vi "OAT Even Angle Signal Subset (1 Channel).vi"(0 "even-angle signal":cluster{"r0":dbl, "dr":dbl, "Y":dbl[]}={"r0"=0.0, "dr"=1.0, "Y"=[]} {"r0" format="%.2p"; "dr" format="%.2p"; "Y" format="%.2f"}, 5 "even-angle channel info":T1={"channel name"="", "description"="", " channel info"={"sensor sensitivity"=1000.0, "engineering units"=1, "dB reference"=1.0, "custom label"="EU", "weighting filter"=0, "pregain"=0.0}} {"channel info"."pregain" format="%.2f"; "channel info"."weighting filter" items=["Linear", "A-weighting", "B-weighting", "C-weighting", "ITU-R 468-4", "Dolby", "CCITT", "C-message", "Wb", "Wc", "Wd", "We", "Wf", "Wh", "Wj", "Wk", "Wm", "AES17 20 kHz lowpass", "AES17 40 kHz lowpass", "AES17 20 kHz highpass", "AES17 40 kHz highpass"]; "channel info"."dB reference" format="%^.1e"; "channel info"."engineering units" items=["custom..."=0, "V"=1, "A"=21, "C"=30, "pC"=31, "s"=32, "-"=29, "Pa"=2, "N"=20, "g"=3, "m/s^2"=4, "m/s"=5, "m"=6, "mm/s"=12, "mm"=13, "micron/s"=14, "micron"=15, "in/s^2"=7, "in/s"=8, "in"=9, "mil/s"=10, "mil"=11, "rad/s^2"=16, "rad/s"=17, "rad"=18, "deg/s^2"=26, "deg/s"=27, "deg"=28, "RPM"=22, "cycle/s^2"=23, "Hz"=24, "cycle"=25, "strain"=19]; "channel info"."sensor sensitivity" format="%#_5f"}, 7 "start [rev]":dbl format="%0.2f", 9 "duration [rev]":dbl=1.0 format="%0.2f", 11 "error in (no error)":errorcluster) -> (4 "even-angle signal subset":cluster{"r0":dbl, "dr":dbl, "Y":dbl[]}={"r0"=0.0, "dr"=1.0, "Y"=[]} {"r0" format="%.2p"; "dr" format="%.2p"; "Y" format="%.2f"}, 6 "even-angle channel info":T1={"channel name"="", "description"="", " channel info"={"sensor sensitivity"=1000.0, "engineering units"=1, "dB reference"=1.0, "custom label"="EU", "weighting filter"=0, "pregain"=0.0}} {"channel info"."pregain" format="%.2f"; "channel info"."weighting filter" items=["Linear", "A-weighting", "B-weighting", "C-weighting", "ITU-R 468-4", "Dolby", "CCITT", "C-message", "Wb", "Wc", "Wd", "We", "Wf", "Wh", "Wj", "Wk", "Wm", "AES17 20 kHz lowpass", "AES17 40 kHz lowpass", "AES17 20 kHz highpass", "AES17 40 kHz highpass"]; "channel info"."dB reference" format="%^.1e"; "channel info"."engineering units" items=["custom..."=0, "V"=1, "A"=21, "C"=30, "pC"=31, "s"=32, "-"=29, "Pa"=2, "N"=20, "g"=3, "m/s^2"=4, "m/s"=5, "m"=6, "mm/s"=12, "mm"=13, "micron/s"=14, "micron"=15, "in/s^2"=7, "in/s"=8, "in"=9, "mil/s"=10, "mil"=11, "rad/s^2"=16, "rad/s"=17, "rad"=18, "deg/s^2"=26, "deg/s"=27, "deg"=28, "RPM"=22, "cycle/s^2"=23, "Hz"=24, "cycle"=25, "strain"=19]; "channel info"."sensor sensitivity" format="%#_5f"}, 15 "error out":errorcluster)   [LabVIEW 2017, in "SoundVib_OAUtility.lvlib"]
doc: "Retrieves a subset of an even-angle signal at a specified revolution duration. This VI does not maintain state internally; you can use this VI in a loop to process multiple blocks. Wire data to the <B>even-angle signal</B> input to determine the polymorphic instance to use or manually select the instance."
uses:
  <vilib>/addons/Sound and Vibration/Order Analysis/Utility/SoundVib_OAUtility.lvlib
  <vilib>/addons/_NISVFA/_Shared subVIs/Controls/svc_Resampled Channel Info.ctl
  <vilib>/addons/_NISVFA/_Shared subVIs/Controls/svc_Channel Info.ctl
  <vilib>/addons/_NISVFA/_Shared subVIs/Controls/svc_Engineering Units Text Ring.ctl
  <vilib>/addons/_NISVFA/_Shared subVIs/Controls/svc_Weighting Filter Text Ring.ctl
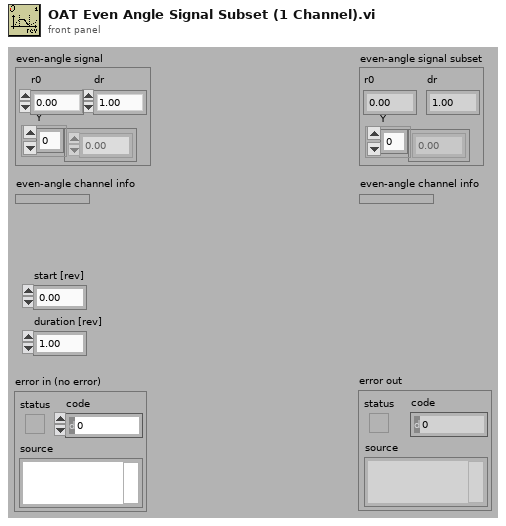
[diagram p1: front panel]
types:
  T1 = typedef "svc_Resampled Channel Info.ctl" = cluster{"channel name":string, "description":string, " channel info":T2}
  T2 = typedef "svc_Channel Info.ctl" = cluster{"sensor sensitivity":dbl, "engineering units":T3, "dB reference":dbl, "custom label":string, "weighting filter":T4, "pregain":dbl}
  T3 = typedef "svc_Engineering Units Text Ring.ctl" = u16
  T4 = typedef "svc_Weighting Filter Text Ring.ctl" = u16
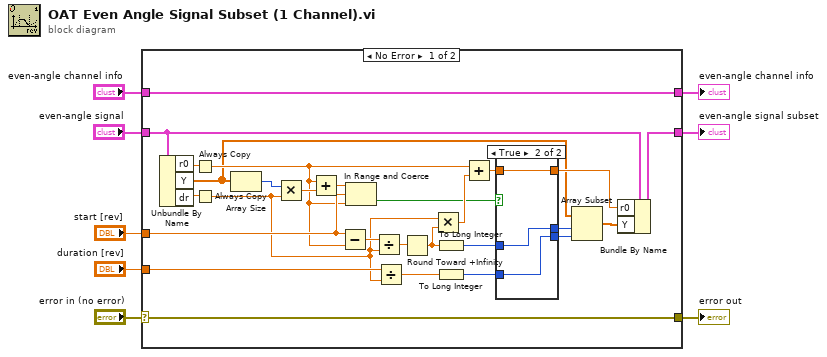
[diagram p0: block diagram]
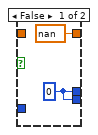
[diagram p2: hidden frame]
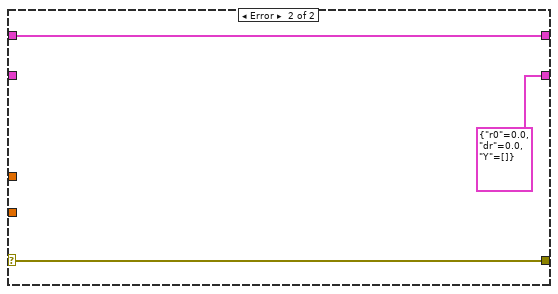
[diagram p3: hidden frame]
diagram:
  n1 = case shown="No Error" "error in (no error)" {
    selector: "error in (no error)" -> [w35 w43]
    tunnel: [w35 w43] -> w7
    tunnel: [w34 w41] -> w6
    tunnel: "even-angle channel info" -> [w34 w41]
    tunnel: "even-angle signal" -> [w29 _]
    tunnel: "start [rev]" -> [w30 _]
    tunnel: "duration [rev]" -> [w28 _]
    tunnel: [w23 cluster{"r0":dbl, "dr":dbl, "Y":dbl[]} {"r0"=0.0, "dr"=0.0, "Y"=[]} ("even angle signal")] -> w1
    frame No Error {
      n2 = Unbundle By Name(w29) -> ("r0"=w22:dbl, "Y"=w9:dbl[], "dr"=w21:dbl)
      n3 = Always Copy(1:w22) -> (0:w18:dbl)
      n4 = Always Copy(1:w21) -> (0:w17:dbl)
      n5 = Array Size(array=w9) -> (size(s)=w33:i32)
      n6 = Multiply(x=w33, y=w17) -> (x*y=w32:dbl)
      n7 = Add(x=w18, y=w32) -> (x+y=w31:dbl)
      n8 = Subtract(x=w30, y=w18) -> (x-y=w27:dbl)
      n9 = In Range and Coerce(upper limit=w31, x=w30, lower limit=w18) -> (In Range?=w16:bool)  [unwired: 1 out]
      n10 = Divide(x=w27, y=w17) -> (x/y=w26:dbl)
      n11 = Divide(x=w28, y=w17) -> (x/y=w19:dbl)
      n12 = Round Toward +Infinity(x=w26) -> (ceil(x): smallest int >= x=w20:dbl)
      n13 = Multiply(x=w17, y=w20) -> (x*y=w25:dbl)
      n14 = To Long Integer(number=w20) -> (32bit integer=w13:i32)
      n15 = To Long Integer(number=w19) -> (32bit integer=w11:i32)
      n16 = Add(x=w18, y=w25) -> (x+y=w15:dbl)
      n17 = case shown="True" w16 {
        tunnel: w15 -> [_ w40]
        tunnel: [nan w40] -> w14
        tunnel: w13 -> [_ w39]
        tunnel: [w36 w39] -> w12
        tunnel: w11 -> [_ w38]
        tunnel: [w36 w38] -> w10
        frame False {
          w36 = 0
        }
        frame True {
        }
      }
      n18 = Array Subset(array=w9, index=w12, length=w10) -> (w24:dbl[])
      n19 = Bundle By Name(cluster=w29, "r0"=w14, "Y"=w24) -> (w23:cluster{"r0":dbl, "dr":dbl, "Y":dbl[]})
    }
    frame Error {
    }
  }
  "error out" <- w7
  "even-angle signal subset" <- w1
  "even-angle channel info" <- w6
